vi "Reponse length.vi"() -> (1 "headers length include length":i32, 3 "headers length":i32)   [LabVIEW 2019]
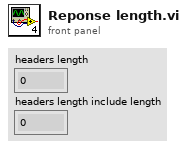
[diagram p1: front panel]
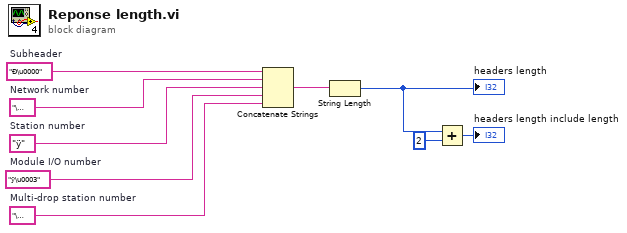
[diagram p0: block diagram]
diagram:
  w5 = "\u0000"  # Multi-drop station number
  w6 = "ÿ\u0003"  # Module I/O number
  w7 = "ÿ"  # Station number
  w8 = "\u0000"  # Network number
  w9 = "Ð\u0000"  # Subheader
  n1 = Concatenate Strings(w9, w8, w7, w6, w5) -> (w4:string)
  n2 = String Length(string=w4) -> (length=w2:i32)
  "headers length" <- w2
  n3 = Add(x=w2, y=2) -> (x+y=→"headers length include length":i32)
